vi "Testing png.vi"(4 "bottom":i16, 6 "top":i16, 7 "Jump Table":dbl[](array[numeric]), 8 "error in":errorcluster, 9 "Doodle in":T2, 10 "background":picture, 11 "FPGA VI Reference In":T1) -> (0 "error out":errorcluster, 3 "FPGA VI Reference Out":T1)   [LabVIEW 2019]
uses:
  <vilib>/picture/picture.llb/imagedata.ctl
  TypeDefs/FPGA Reference.ctl
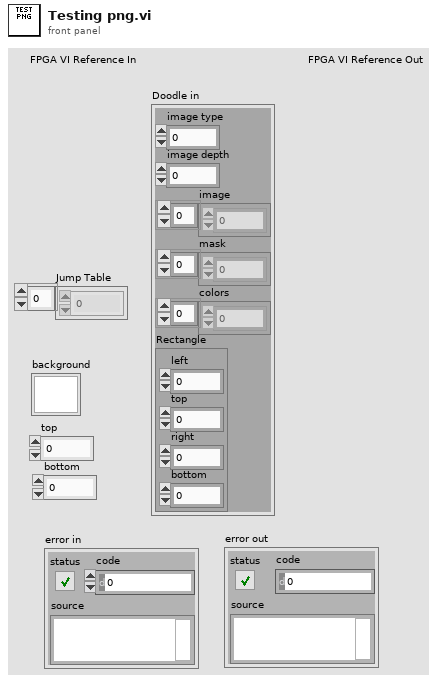
[diagram p1: front panel]
types:
  T1 = typedef "FPGA Reference.ctl" = refnum<k20>
  T2 = typedef "imagedata.ctl" = cluster{"image type":i32, "image depth":i32, "image":u8[], "mask":u8[], "colors":u32[], "Rectangle":cluster{"left":i16, "top":i16, "right":i16, "bottom":i16}}
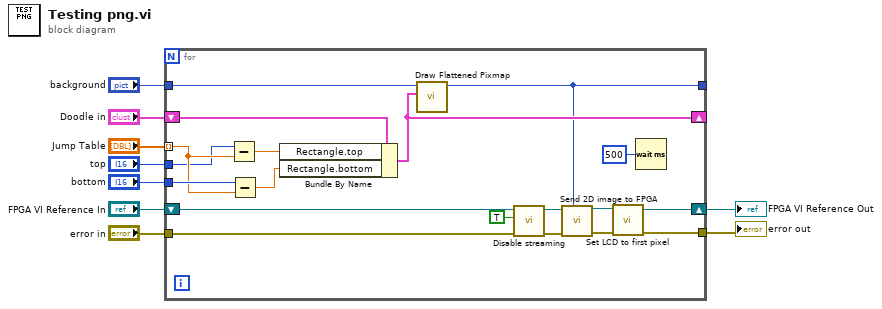
[diagram p0: block diagram]
diagram:
  n1 = for {
    tunnel: "Jump Table" -> [w23] mode=indexing
    tunnel: "top" -> [w22]
    tunnel: "bottom" -> [w24]
    shift-right: [w25] -> _
    shift-left: "Doodle in" -> [w28]
    tunnel: "background" -> [w12]
    tunnel: [w11] -> _
    tunnel: "error in" -> [w18]
    tunnel: [w17] -> w2
    shift-right: [w15] -> w1
    shift-left: "FPGA VI Reference In" -> [w20]
    n2 = Subtract(x=w22, y=w23) -> (x-y=w27:dbl)
    n3 = Subtract(x=w24, y=w23) -> (x-y=w26:dbl)
    n4 = Bundle By Name(cluster=w28, "Rectangle.top"=w27, "Rectangle.bottom"=w26) -> (w25:T2)
    n5 = call <vilib>:"Draw Flattened Pixmap.vi"("image data"=w25, "picture"=w12) -> ("new picture"=w11:picture)  [unwired: 7 in]
    n6 = call "Disable streaming.vi"("error in"=w18, "StreamDisabled"=TRUE, "FPGA VI Reference Out"=w20) -> ("error out"=w14:errorcluster, "FPGA VI Reference Out 2"=w21:T1)  [unwired: 7 in]
    n7 = call "Send 2D image to FPGA.vi"("picture"=w11, "error in"=w14, "FPGA VI Reference Out"=w21) -> ("error out"=w13:errorcluster, "FPGA VI Reference Out 2"=w19:T1)  [unwired: 7 in]
    n8 = call "Set LCD to first pixel.vi"("error in"=w13, "FPGA VI Reference In"=w19) -> ("error out"=w17:errorcluster, "FPGA VI Reference Out"=w15:T1)  [unwired: 8 in]
    n9 = Wait (ms)(milliseconds to wait=u32 500) -> ()  [unwired: 1 out]
  }
  "error out" <- w2
  "FPGA VI Reference Out" <- w1
